vi "forward_kinematics.vi"(10 "Axis positions":dbl[](array[numeric]) format="%#.3f") -> (2 "Pose":T1 format="%#_3p")   [LabVIEW 2012]
uses:
  <vilib>/Analysis/Matrix/Datatypes/RealMatrix.ctl
  <vilib>/Analysis/coordinate.llb/Euler Rotation Order.ctl
  <vilib>/Analysis/Matrix/Numeric/Conversions/Array To Matrix - RA.vi
  <vilib>/Analysis/baseanly.llb/Real A x B.vi
  <vilib>/Analysis/NI_AALBase.lvlib
  <vilib>/Analysis/Matrix/NI_Matrix.lvlib
  <vilib>/Analysis/NI_AALPro.lvlib
panel:
  # "Find the forward kinematics of the motion stage: the output pose resulting from specified axis positions."
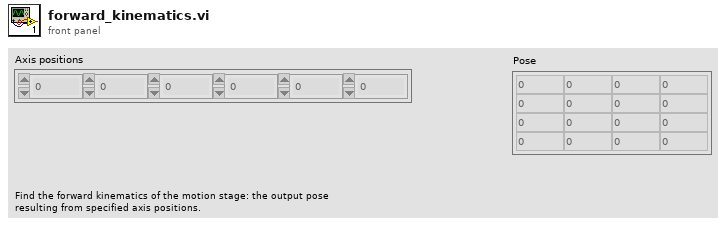
[diagram p1: front panel]
types:
  T1 = typedef "NI_Matrix.lvlib/RealMatrix.ctl" = dbl[][]
  T2 = typedef "NI_AALPro.lvlib/Euler Rotation Order.ctl" = u16
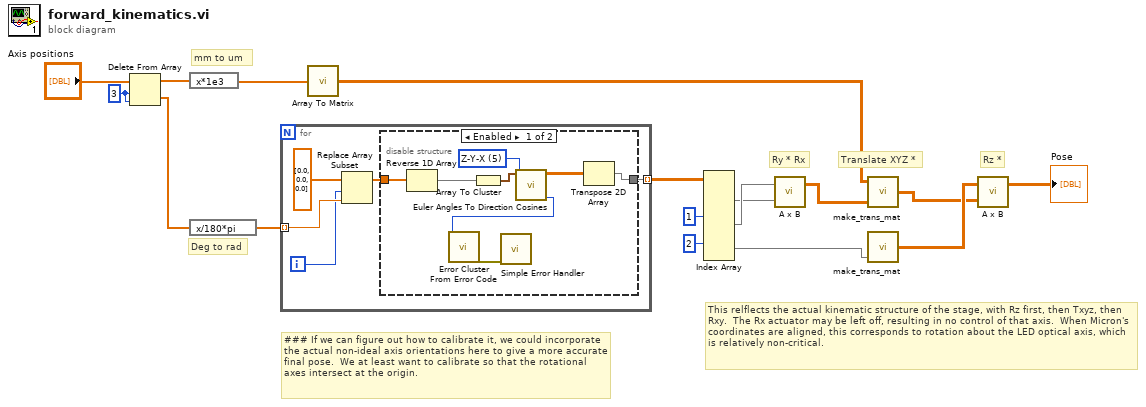
[diagram p0: block diagram]
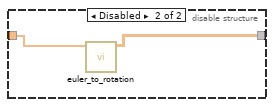
[diagram p2: hidden frame]
diagram:
  w17 = 3 ("length")
  # "This relflects the actual kinematic structure of the stage, with Rz first, then Txyz, then Rxy.  The Rx actuator may be left off, resulting in no control of that axis.  When Micron's coordinates are aligned, this corresponds to rotation about the LED optical axis, which is relatively non-critical."
  # "Rz *"
  # "Translate XYZ *"
  # "Ry * Rx"
  # "### If we can figure out how to calibrate it, we could incorporate the actual non-ideal axis orientations here to give a more accurate final pose.  We at least want to calibrate so that the rotational axes intersect at the origin."
  # "mm to um"
  # "Deg to rad"
  n1 = Delete From Array(array="Axis positions", length=w17, index=w17) -> (deleted portion=w16:dbl[], array with subset deleted=w15:dbl[])
  n2 = expression code="x*1e3"(w15) -> (w7:dbl[])
  n3 = expression code="x/180*pi"(w16) -> (w12:dbl[])
  n4 = for {
    tunnel: w12 -> [w22] mode=indexing
    tunnel: [w18] -> w11 mode=indexing
    i -> [w20]
    n5 = Replace Array Subset(array=dbl[] [0.0, 0.0, 0.0], new element=w22, index=w20) -> (w19:dbl[])
    n6 = disable-structure shown="Enabled" {
      disable-tunnel: w19 -> [w26 w32]
      disable-tunnel: [w23 w31] -> w18
      frame Enabled {
        w27 = T2 5 items=["X-Y-Z", "X-Z-Y", "Y-X-Z", "Y-Z-X", "Z-X-Y", "Z-Y-X", "X-Y-X", "X-Z-X", "Y-X-Y", "Y-Z-Y", "Z-X-Z", "Z-Y-Z"] ("rotation order")
        n7 = Reverse 1D Array(array=w26) -> (reversed array=w25:dbl[])
        n8 = Array To Cluster(array=w25) -> (cluster=w30:cluster{"[0]":dbl, "[1]":dbl, "[2]":dbl})
        n9 = call <vilib>:"Euler Angles To Direction Cosines.vi"("rotation order"=w27, "Euler Angles"=w30) -> ("error"=w29:i32, "Direction Cosines"=w24:dbl[][])  [unwired: 8 in]
        n10 = call <vilib>:"Error Cluster From Error Code.vi"("error code (0)"=w29) -> ("error out"=w28:errorcluster)  [unwired: 8 in]
        n11 = call <vilib>:"Simple Error Handler.vi"("error in (no error)"=w28) -> ()  [unwired: 4 in, 5 out]
        n12 = Transpose 2D Array(2D array=w24) -> (transposed array=w23:dbl[][])
      }
      frame Disabled {
        n13 = call "euler_to_rotation.vi"("Theta XYZ"=w32) -> ("Rotation"=w31:T1)  [unwired: 10 in]
      }
    }
  }
  n14 = call-poly <vilib>:"Array To Matrix.vi"("Real 1D Array"=w7) -> ("Real Matrix (Column Vector)"=w6:T1)
  n15 = Index Array(array=w11, index (dim 0) #2=1 ("index"), index (dim 0) #3=2 ("index")) -> (element #1=w9:dbl[][], element #2=w10:dbl[][], element #3=w4:dbl[][])  [unwired: 7 in]
  n16 = call-poly <vilib>:"A x B.vi"("B"=w9, "A"=w10) -> ("A x B"=w8:T1)  [unwired: 1 out]
  n17 = call "make_trans_mat.vi"("Rotation"=w8, "Translation"=w6) -> ("Transform"=w2:T1)  [unwired: 3 in]
  n18 = call "make_trans_mat.vi"("Rotation"=w4) -> ("Transform"=w3:T1)  [unwired: 4 in]
  n19 = call-poly <vilib>:"A x B.vi"("B"=w2, "A"=w3) -> ("A x B"=→"Pose":T1)  [unwired: 1 out]
